vi "ATT Driver.vi"(5 "ATT Configuration (\"\")":string, 6 "Drv Refnum":T1, 7 "ATT Command":T2, 8 "error in (no error)":errorcluster, 10 "ATT Value In":T3={"Normalize"=TRUE, "Value (dB)"=0.0}) -> (0 "error out":errorcluster, 1 "ATT Flat Output":string, 2 "ATT Value Out":T3={"Normalize"=TRUE, "Value (dB)"=0.0}, 4 "dup Drv Refnum":T1)   [LabVIEW 2011]
uses:
  tests/Attenuator/TypeDefs/Attenuator ATT Stimulus.ctl
  ATT Command.ctl
  ATT Driver Ref.ctl
panel:
  in  "DEBUG?":bool
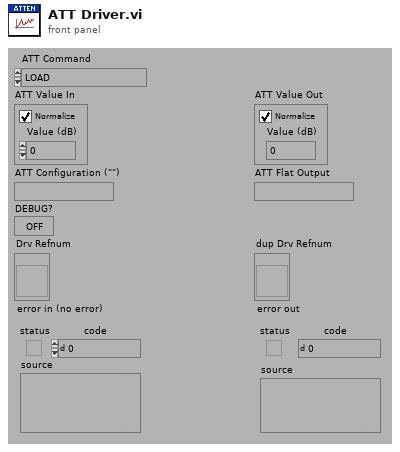
[diagram p1: front panel]
types:
  T1 = typedef "ATT Driver Ref.ctl" = refnum<vi>
  T2 = typedef "ATT Command.ctl" = enum16{"LOAD", "INITIALIZE", "PRESET", "SET STIMULUS", "GET STIMULUS", "GET CALIBRATION", "CALIBRATE", "GET INFO", "RELEASE", "UNLOAD"}
  T3 = typedef "Attenuator ATT Stimulus.ctl" = cluster{"Normalize":bool, "Value (dB)":dbl}
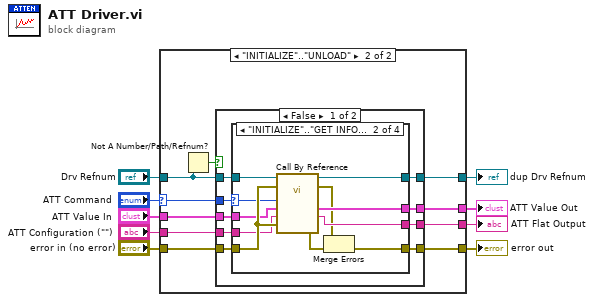
[diagram p0: block diagram]
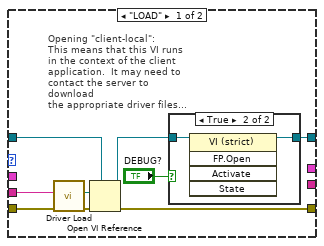
[diagram p2: hidden frame]
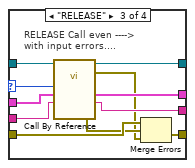
[diagram p5: hidden frame]
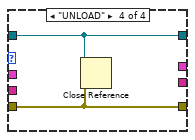
[diagram p6: hidden frame]
diagram:
  n1 = case shown="\"INITIALIZE\"..\"UNLOAD\"" "ATT Command" {
    selector: "ATT Command" -> [_ w24]
    tunnel: "error in (no error)" -> [w18 w31]
    tunnel: "ATT Value In" -> [_ w30]
    tunnel: [_ w29] -> w7
    tunnel: [w17 w28] -> w6
    tunnel: "ATT Configuration (\"\")" -> [w16 w27]
    tunnel: [_ w26] -> w4
    tunnel: [w15 w25] -> w3
    tunnel: "Drv Refnum" -> [w14 w23]
    frame "LOAD" {
      # "Opening \"client-local\":\nThis means that this VI runs\nin the context of the client\napplication.  It may need to\ncontact the server to download\nthe appropriate driver files..."
      n2 = call "Driver Load.vi"("error in (no error)"=w18, "DriverID DriverType (\"\")"=w16) -> ("error out"=w10:errorcluster, "Driver Component Path"=w11:path)  [unwired: 1 in, 7 out]
      n3 = Open VI Reference(type specifier VI Refnum (for type only)=w14, vi path=w11, error in (no error)=w10) -> (vi reference=w13:T1, error out=w17:errorcluster)  [unwired: 3 out]
      n4 = case shown="True" "DEBUG?" {
        tunnel: w13 -> [w19 w21]
        tunnel: [w19 w20] -> w15
        frame False {
        }
        frame True {
          n5 = invoke class="VI (strict)" method="FP.Open"(reference=w21) -> (reference out=w20:T1)  [unwired: 4 in, 4 out]
        }
      }
    }
    frame "INITIALIZE".."UNLOAD" {
      n6 = Not A Number/Path/Refnum?(number/path/refnum=w23) -> (NaN/Path/Refnum?=w22:bool)
      n7 = case shown="False" w22 {
        tunnel: w31 -> [w40 w67]
        tunnel: w30 -> [w39 _]
        tunnel: [w38 _] -> w29
        tunnel: [w37 w67] -> w28
        tunnel: w27 -> [w36 _]
        tunnel: [w35 _] -> w26
        tunnel: [w34 w68] -> w25
        tunnel: w23 -> [w33 w68]
        tunnel: w24 -> [w32 _]
        frame False {
          n8 = case shown="\"INITIALIZE\"..\"GET INFO\"" w32 {
            selector: w32 -> [_ w45 w60 _]
            tunnel: w40 -> [w42 w51 w58 w65]
            tunnel: w39 -> [_ w43 w54 _]
            tunnel: [_ w50 w62 _] -> w38
            tunnel: [w42 w53 w64 w65] -> w37
            tunnel: w36 -> [_ w48 w59 _]
            tunnel: [_ w49 w61 _] -> w35
            tunnel: [w41 w52 w63 w66] -> w34
            tunnel: w33 -> [w41 w44 w55 w66]
            frame "LOAD", Default {
              # "This will not ever run."
            }
            frame "INITIALIZE".."GET INFO" {
              n9 = call-by-ref "?"(reference=w44, error in=w51, "error in (no error)"=w51, "ATT Configuration (\"\")"=w48, "ATT Value In"=w43, "ATT Command"=w45) -> (reference out=w52:T1, error out=w46:errorcluster, 0:"error out"=w47:errorcluster, "ATT Flat Output"=w49:string, "ATT Value Out"=w50:T3)  [unwired: 5 in]
              n10 = Merge Errors(w46, w47) -> (w53:errorcluster)
            }
            frame "RELEASE" {
              # "RELEASE Call even ---->\nwith input errors...."
              n11 = call-by-ref "?"(reference=w55, "ATT Configuration (\"\")"=w59, "ATT Value In"=w54, "ATT Command"=w60) -> (reference out=w63:T1, error out=w56:errorcluster, 0:"error out"=w57:errorcluster, "ATT Flat Output"=w61:string, "ATT Value Out"=w62:T3)  [unwired: 7 in]
              n12 = Merge Errors(w58, w57, w56) -> (w64:errorcluster)
            }
            frame "UNLOAD" {
              n13 = Close Reference(reference=w66, error in (no error)=w65) -> ()  [unwired: 1 out]
            }
          }
        }
        frame True {
          # "If the reference is not valid\nno operation is performed."
        }
      }
    }
  }
  "error out" <- w6
  "ATT Value Out" <- w7
  "ATT Flat Output" <- w4
  "dup Drv Refnum" <- w3
